vi "CastArrayDependenciesToClusterOrClass.vi"(7 "Dependency Type (Class|Cluster)":variant, 8 "error in (no error)":errorcluster, 10 "index (-1: from start)":i32=-1, 11 "[Dependencies]":refnum<class>[](array[class])) -> (0 "error out":errorcluster, 3 "Dependencies output":variant)   [LabVIEW 2013, in "SMO.lvclass"]
uses:
  SMO.lvclass
  <vilib>/Utility/VariantDataType/VariantType.lvlib
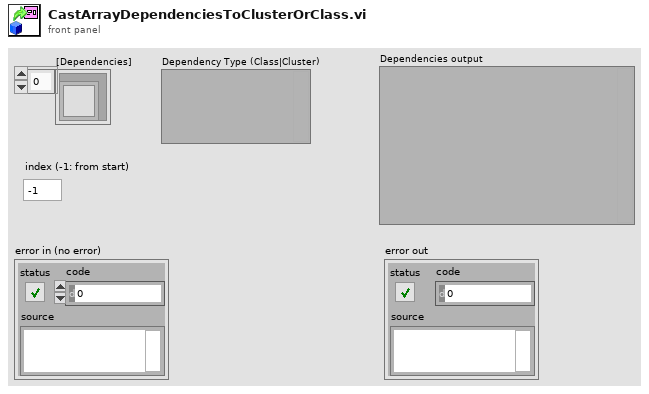
[diagram p1: front panel]
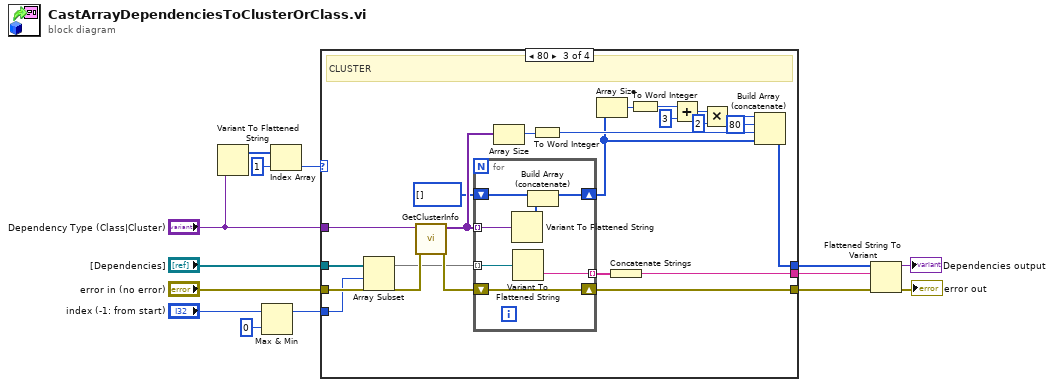
[diagram p0: block diagram]
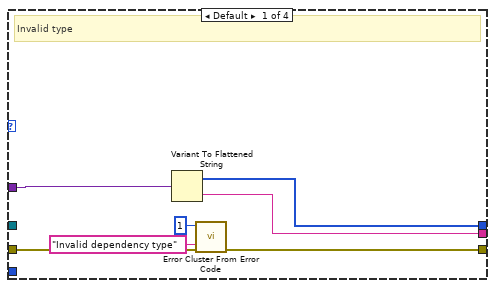
[diagram p2: hidden frame]
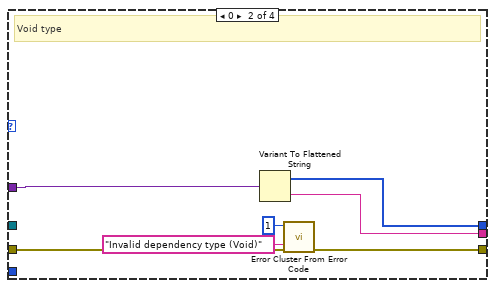
[diagram p3: hidden frame]
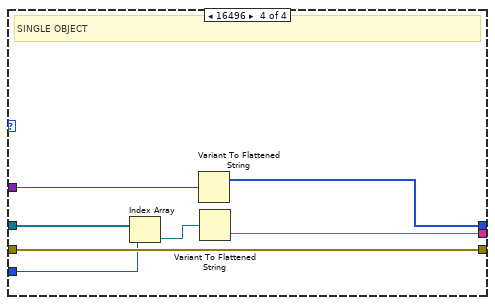
[diagram p4: hidden frame]
diagram:
  n1 = Variant To Flattened String(Variant="Dependency Type (Class|Cluster)") -> (1:w7:i16[])  [unwired: 1 out]
  n2 = Max & Min(x="index (-1: from start)", y=0) -> (max(x,y)=w1:i32)  [unwired: 1 out]
  n3 = Index Array(array=w7, index=1) -> (element=w5:i16)
  n4 = case shown="80" w5 {
    tunnel: [w17 w24 w50 w63] -> w12
    tunnel: "[Dependencies]" -> [_ _ w31 w60]
    tunnel: "error in (no error)" -> [w18 w25 w49 w63]
    tunnel: [w19 w26 w42 w61] -> w9
    tunnel: [w20 w27 w34 w62] -> w8
    tunnel: "Dependency Type (Class|Cluster)" -> [w21 w28 w33 w64]
    tunnel: w1 -> [_ _ w29 w58]
    frame Default {
      # "Invalid type"
      n5 = Variant To Flattened String(Variant=w21) -> (data string=w19:string, 1:w20:i16[])
      n6 = call <vilib>:"Error Cluster From Error Code.vi"("error in (no error)"=w18, "error message (\"\")"="Invalid dependency type" ("error message (\"\")"), "error code (0)"=1) -> ("error out"=w17:errorcluster)  [unwired: 6 in]
    }
    frame 0 {
      # "Void type"
      n7 = Variant To Flattened String(Variant=w28) -> (data string=w26:string, 1:w27:i16[])
      n8 = call <vilib>:"Error Cluster From Error Code.vi"("error in (no error)"=w25, "error message (\"\")"="Invalid dependency type (Void)" ("error message (\"\")"), "error code (0)"=1) -> ("error out"=w24:errorcluster)  [unwired: 6 in]
    }
    frame 80 {
      # "CLUSTER"
      n9 = Array Subset(array=w31, index=w29) -> (w30:refnum<class>[])  [unwired: 1 in]
      n10 = call <vilib>:"GetClusterInfo.vi"("error in (no error)"=w49, "Variant"=w33) -> ("error out"=w48:errorcluster, "Cluster Elements"=w47:variant[])  [unwired: 8 in]
      n11 = for {
        tunnel: w30 -> [w57] mode=indexing
        shift-right: [w56] -> w50
        shift-left: w48 -> [w56]
        tunnel: w47 -> [w55] mode=indexing
        shift-right: [w53] -> w35
        shift-left: i16[] [] -> [w54]
        tunnel: [w52] -> w43 mode=indexing
        n12 = Variant To Flattened String(Variant=w55) -> (1:w51:i16[])  [unwired: 1 out]
        n13 = Variant To Flattened String(Variant=w57) -> (data string=w52:string)  [unwired: 1 out]
        n14 = Build Array (concatenate)(w54, w51) -> (w53:i16[])
      }
      n15 = Array Size(array=w47) -> (size(s)=w46:i32)
      n16 = To Word Integer(number=w46) -> (16bit integer=w45:i16)
      n17 = Array Size(array=w35) -> (size(s)=w37:i32)
      n18 = Concatenate Strings(w43) -> (w42:string)
      n19 = To Word Integer(number=w37) -> (16bit integer=w41:i16)
      n20 = Add(x=w41, y=i16 3) -> (x+y=w39:i16)
      n21 = Multiply(x=w39, y=i16 2) -> (x*y=w36:i16)
      n22 = Build Array (concatenate)(w36, i16 80 ("16bit integer"), w45, w35) -> (w34:i16[])
    }
    frame 16496 {
      # "SINGLE OBJECT"
      n23 = Index Array(array=w60, index=w58) -> (element=w59:refnum<class>)
      n24 = Variant To Flattened String(Variant=w64) -> (1:w62:i16[])  [unwired: 1 out]
      n25 = Variant To Flattened String(Variant=w59) -> (data string=w61:string)  [unwired: 1 out]
    }
  }
  n26 = Flattened String To Variant(4:w12, 6:w9, 7:w8) -> (0:→"error out":errorcluster, 3:→"Dependencies output":variant)
